vi "set_legend_names.vi"(7 "appended array":bool[](array[boolean]), 11 "Input Plot Ref":refnum<vi>) -> ()   [LabVIEW 2020]
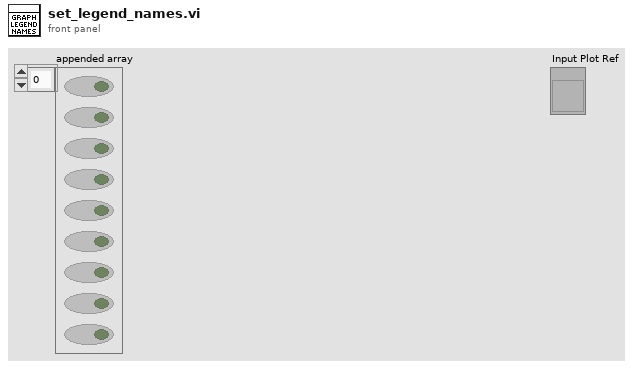
[diagram p1: front panel]
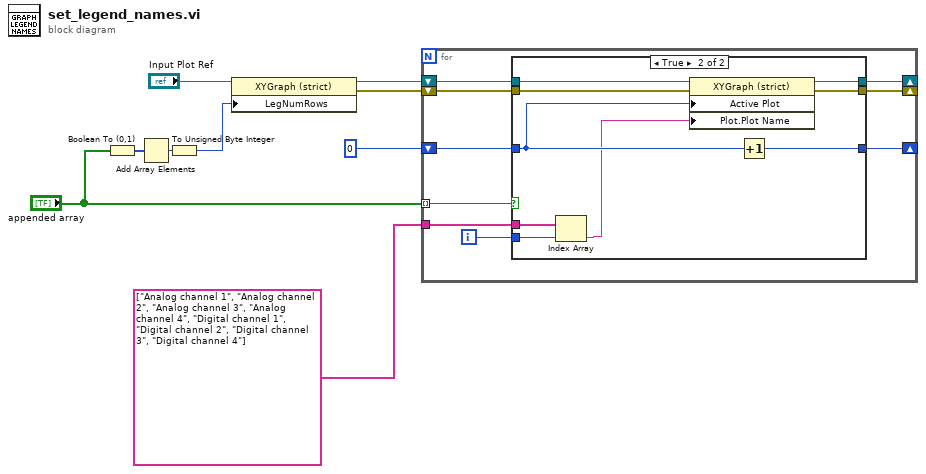
[diagram p0: block diagram]
diagram:
  n1 = Boolean To (0,1)(Boolean="appended array") -> (0, 1=w5:i16[])
  n2 = Add Array Elements(numeric array=w5) -> (sum=w6:i16)
  n3 = To Unsigned Byte Integer(number=w6) -> (unsigned 8bit integer=w3:u8)
  n4 = property class="XYGraph (strict)"(reference="Input Plot Ref", "LegNumRows"=w3) -> (reference out=w9:refnum<vi>, error out=w8:errorcluster)  [unwired: 1 in]
  n5 = for {
    tunnel: "appended array" -> [w14] mode=indexing
    shift-right: [w15] -> _
    shift-left: w8 -> [w17]
    shift-right: [w16] -> _
    shift-left: w9 -> [w18]
    shift-right: [w12] -> _
    shift-left: u32 0 ("Active Plot") -> [w13]
    tunnel: string[] ["Analog channel 1", "Analog channel 2", "Analog channel 3", "Analog channel 4", "Digital channel 1", "Digital channel 2", "Digital channel 3", "Digital channel 4"] -> [w11]
    i -> [w10]
    n6 = case shown="True" w14 {
      tunnel: w18 -> [w21 w30]
      tunnel: w17 -> [w20 w29]
      tunnel: [w21 w28] -> w16
      tunnel: [w20 w27] -> w15
      tunnel: w13 -> [w19 w26]
      tunnel: [w19 w25] -> w12
      tunnel: w11 -> [_ w24]
      tunnel: w10 -> [_ w23]
      frame False {
      }
      frame True {
        n7 = Index Array(array=w24, index=w23) -> (element=w22:string)
        n8 = property class="XYGraph (strict)"(reference=w30, error in=w29, "Active Plot"=w26, "Plot.Plot Name"=w22) -> (reference out=w28:refnum<vi>, error out=w27:errorcluster)
        n9 = Increment(x=w26) -> (x+1=w25:u32)
      }
    }
  }
